vi "读取-报警文件清单.vi"(11 "报警记录清单":path) -> (0 "报警记录-索引映射":i32[](array[numeric]), 2 "路径数组":string[][](array[string]), 3 "报警列表数组":string[][](array[string]))   [LabVIEW 2013]
uses:
  <vilib>/Utility/file.llb/Read From Spreadsheet File (string).vi
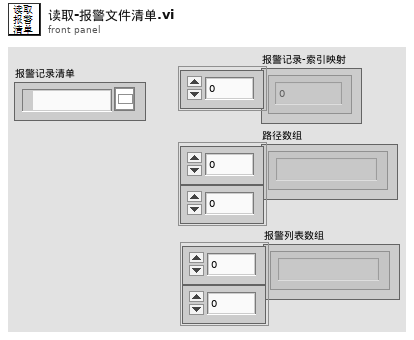
[diagram p1: front panel]
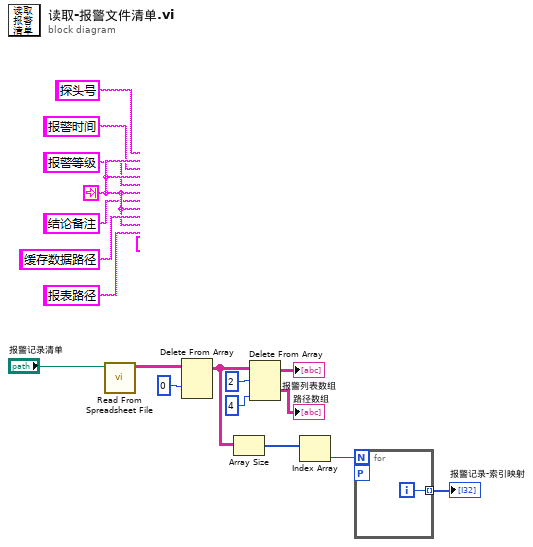
[diagram p0: block diagram]
diagram:
  n1 = call-poly <vilib>:"Read From Spreadsheet File.vi"("file path (dialog if empty)"="报警记录清单") -> ("all rows"=w10:string[][])  [unwired: 6 in, 4 out]
  n2 = Delete From Array(array=w10, index (row)=0 ("索引 (行)")) -> (array with subset deleted=w8:string[][])  [unwired: 2 in, 1 out]
  n3 = Array Size(array=w8) -> (size(s)=w7:i32[])
  n4 = Delete From Array(array=w8, length=2 ("长度"), index (col)=4 ("禁用的索引 (列)")) -> (deleted portion=→"路径数组":string[][], array with subset deleted=→"报警列表数组":string[][])  [unwired: 1 in]
  n5 = Index Array(array=w7) -> (element=w6:i32)  [unwired: 1 in]
  n6 = for {
    N: w6 -> [_]
    workers-P: _ -> [_]
    tunnel: [w12] -> w5 mode=indexing
    i -> [w12]
  }
  "报警记录-索引映射" <- w5
